vi "Counter.vi"(0 "T0":bool, 1 "T4":bool, 5 "T1":bool, 9 "T2":bool, 11 "T3":bool, 12 "clock":bool, 14 "T5":bool) -> (3 "A0":bool, 4 "A1":bool, 6 "A2":bool, 8 "A4":bool, 10 "A3":bool, 15 "A5\nA5":bool)   [LabVIEW 2018]
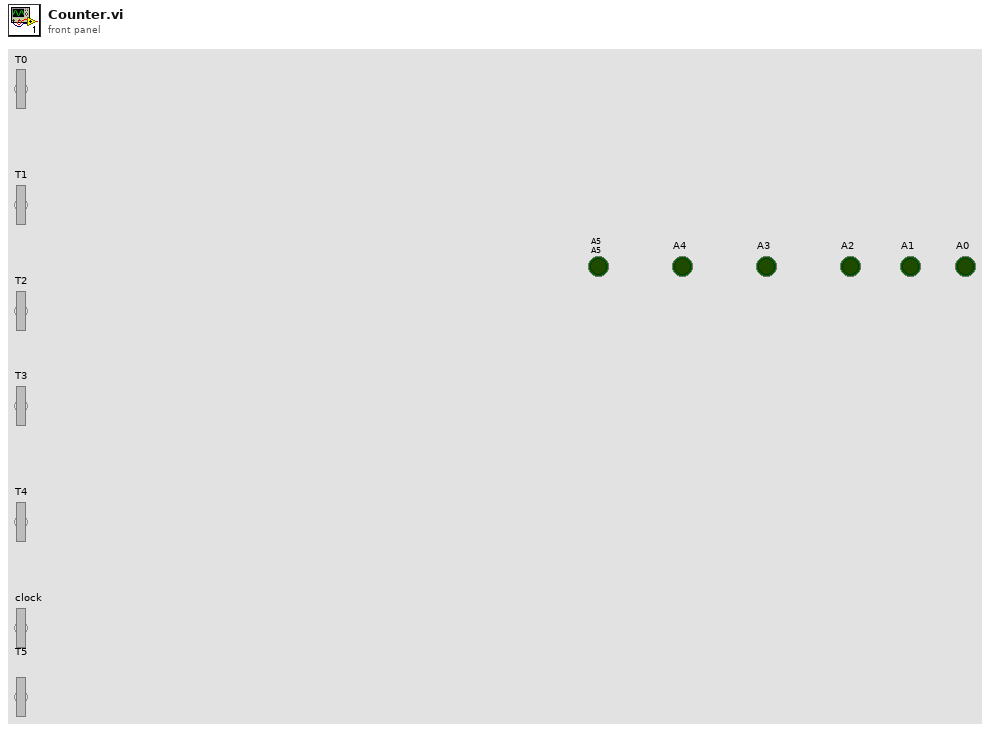
[diagram p1: front panel]
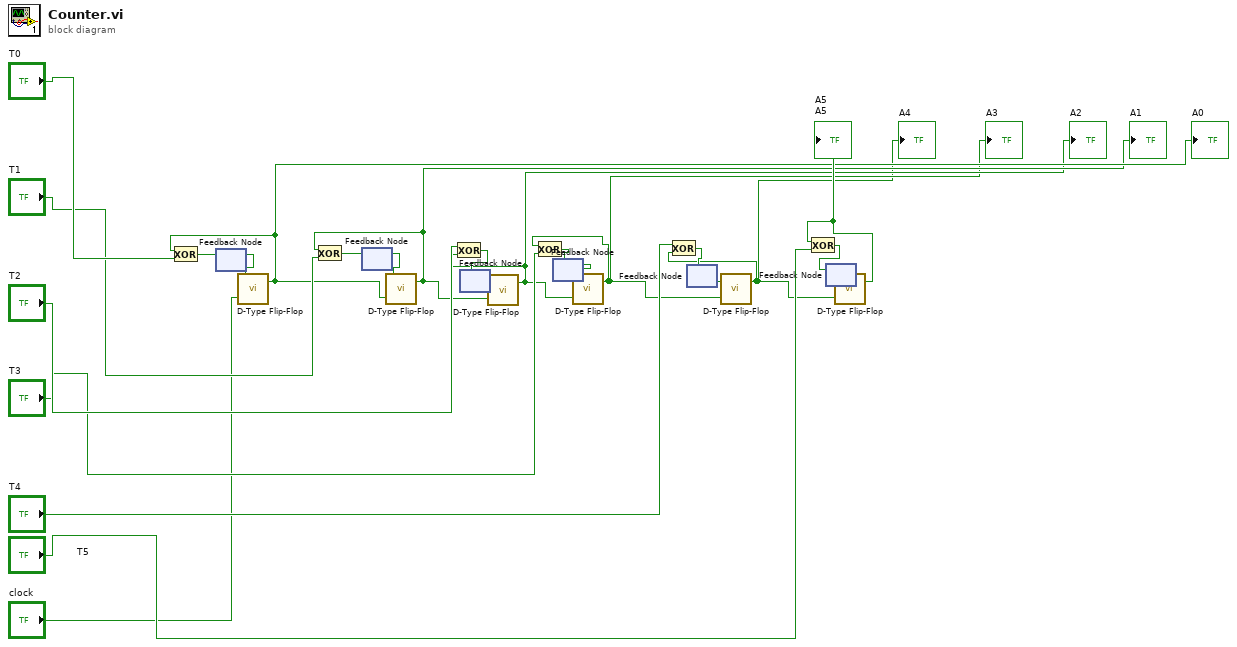
[diagram p0: block diagram]
diagram:
  n1 = feedback #1() -> (w18:bool)  [unwired: 1 in]
  n2 = call "D-Type Flip-Flop.vi"("clock"="clock", "Data"=w18) -> ("Q"=w5:bool)  [unwired: 1 out]
  "A0" <- w5
  n3 = Exclusive Or(1:"T0", 2:w5) -> (0:w19:bool)
  n4 = feedback-in #1(w19) -> ()
  n5 = feedback #2() -> (w16:bool)  [unwired: 1 in]
  n6 = call "D-Type Flip-Flop.vi"("clock"=w5, "Data"=w16) -> ("Q"=w4:bool)  [unwired: 1 out]
  "A1" <- w4
  n7 = Exclusive Or(1:"T1", 2:w4) -> (0:w17:bool)
  n8 = feedback-in #2(w17) -> ()
  n9 = feedback #3() -> (w14:bool)  [unwired: 1 in]
  n10 = call "D-Type Flip-Flop.vi"("clock"=w4, "Data"=w14) -> ("Q"=w3:bool)  [unwired: 1 out]
  "A2" <- w3
  n11 = Exclusive Or(1:w3, 2:"T2") -> (0:w15:bool)
  n12 = feedback-in #3(w15) -> ()
  n13 = feedback #4() -> (w12:bool)  [unwired: 1 in]
  n14 = call "D-Type Flip-Flop.vi"("clock"=w3, "Data"=w12) -> ("Q"=w2:bool)  [unwired: 1 out]
  "A3" <- w2
  n15 = Exclusive Or(1:"T3", 2:w2) -> (0:w13:bool)
  n16 = feedback-in #4(w13) -> ()
  n17 = feedback #5() -> (w10:bool)  [unwired: 1 in]
  n18 = call "D-Type Flip-Flop.vi"("clock"=w2, "Data"=w10) -> ("Q"=w1:bool)  [unwired: 1 out]
  "A4" <- w1
  n19 = Exclusive Or(1:w1, 2:"T4") -> (0:w11:bool)
  n20 = feedback-in #5(w11) -> ()
  n21 = feedback #6() -> (w8:bool)  [unwired: 1 in]
  n22 = call "D-Type Flip-Flop.vi"("clock"=w1, "Data"=w8) -> ("Q"=w6:bool)  [unwired: 1 out]
  "A5\nA5" <- w6
  n23 = Exclusive Or(1:"T5", 2:w6) -> (0:w9:bool)
  n24 = feedback-in #6(w9) -> ()
